vi "Update.vi"(8 "error in (no error)":errorcluster, 11 "HighscoreDialog in":refnum<class "HighscoreDialog.lvclass">) -> (0 "error out":errorcluster, 3 "HighscoreDialog out":refnum<class "HighscoreDialog.lvclass">)   [LabVIEW 2019, in "RT_Game.lvlib" / "HighscoreDialog.lvclass"]
uses:
  HighscoreDialog.lvclass
  GameObject/GameObject.lvclass
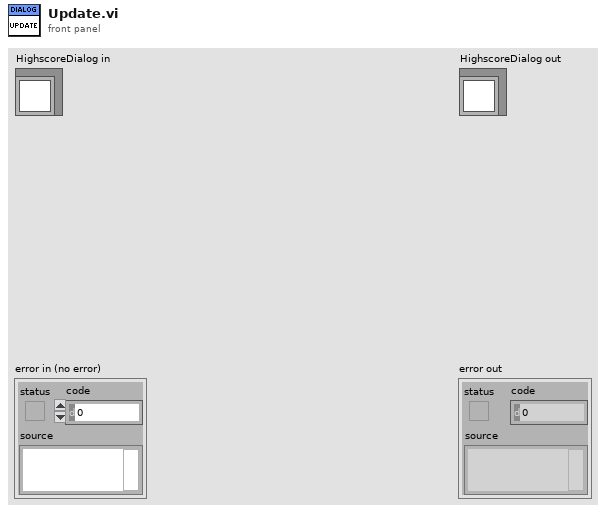
[diagram p1: front panel]
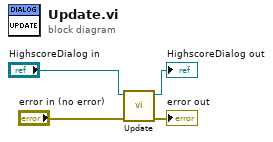
[diagram p0: block diagram]
diagram:
  n1 = call-parent "Update.vi"("error in (no error)"="error in (no error)", "GameObject in"="HighscoreDialog in") -> ("error out"=→"error out":errorcluster, "GameObject out"=→"HighscoreDialog out":refnum<class "HighscoreDialog.lvclass">)  [unwired: 8 in]
